vi "cursor hpos to column.vi"(2 "Selection Position":cluster{i32, i32}, 3 "Voltage set 0":bool, 4 "subpage":bool, 5 "Display":string[][](array[string])) -> (0 "column num":i32, 1 "Column":string)   [LabVIEW 2018]
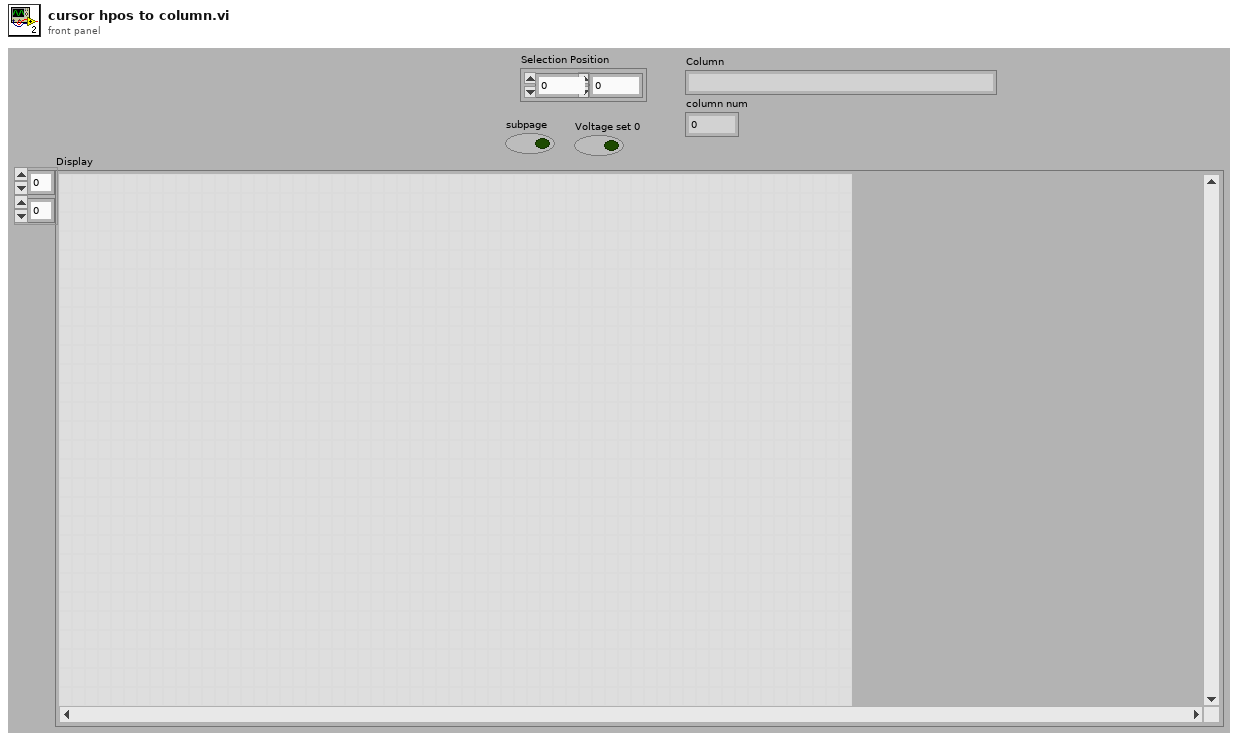
[diagram p1: front panel]
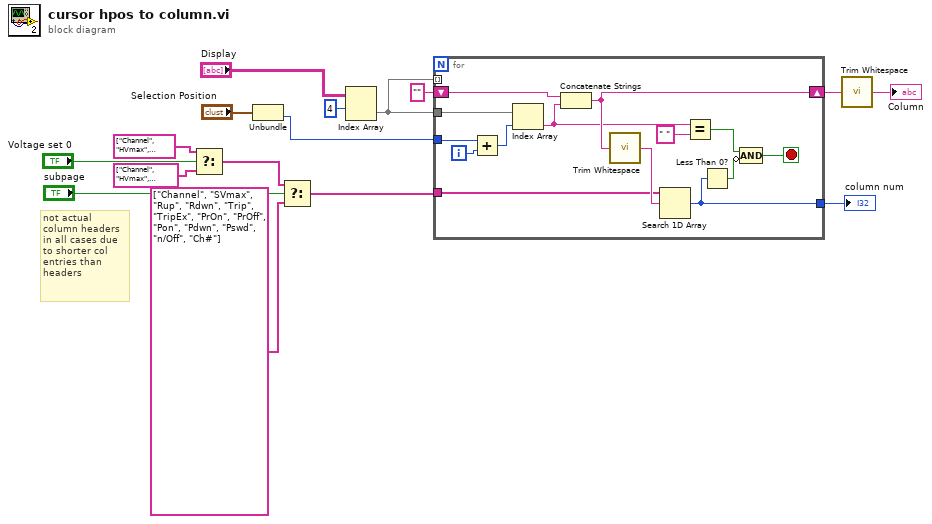
[diagram p0: block diagram]
diagram:
  # "not actual\ncolumn headers\nin all cases due\nto shorter col\nentries than\nheaders"
  n1 = Select(t=string[] ["Channel", "HVmax", "Vmon", "Imon", "V0set", "I0set", "Pw", "Status", "Ch#"] ("subarray"), s="Voltage set 0", f=string[] ["Channel", "HVmax", "Vmon", "Imon", "V1set", "I1set", "Pw", "Status", "Ch#"] ("subarray")) -> (s? t:f=w11:string[])
  n2 = Unbundle("Selection Position") -> (w3:i32)  [unwired: 1 out]
  n3 = Select(t=w11, s="subpage", f=string[] ["Channel", "SVmax", "Rup", "Rdwn", "Trip", "TripEx", "PrOn", "PrOff", "Pon", "Pdwn", "Pswd", "n/Off", "Ch#"] ("Column Headers")) -> (s? t:f=w1:string[])
  n4 = Index Array(array="Display", index (row)=4) -> (element=w7:string[])  [unwired: 1 in]
  n5 = for {
    tunnel: w1 -> [w17]
    tunnel: w7 -> [w30]
    tunnel: w3 -> [w28]
    shift-right: [w24] -> w5
    shift-left: "" -> [w27]
    tunnel: [w26] -> w8
    tunnel: w7 -> [_] mode=indexing
    i -> [w29]
    stop <- w18 stop-if-true
    n6 = Add(x=w28, y=w29) -> (x+y=w25:i32)
    n7 = Index Array(array=w30, index=w25) -> (element=w22:string)
    n8 = Concatenate Strings(w27, w22) -> (w24:string)
    n9 = call <vilib>:"Trim Whitespace.vi"("string"=w24) -> ("trimmed string"=w23:string)  [unwired: 1 in]
    n10 = Search 1D Array(1D array=w17, element=w23) -> (index of element=w26:i32)  [unwired: 1 in]
    n11 = Equal?(x=w22, y=" ") -> (x = y?=w20:bool)
    n12 = Less Than 0?(x=w26) -> (x < 0?=w19:bool)
    n13 = Compound Arithmetic op=AND(w20, invert w19) -> (w18:bool)
  }
  "column num" <- w8
  n14 = call <vilib>:"Trim Whitespace.vi"("string"=w5) -> ("trimmed string"=→"Column":string)  [unwired: 1 in]
